vi "Autonomous.vi"   [LabVIEW 2018]
doc: "This VI starts when autonomous period begins, and will automatically be terminated when it ends. You can carry out timed or sensor driven operations directly to I/O or to subsystems without needing to return to the caller."
uses:
  <vilib>/Rock Robotics/WPI/Solenoid/WPI_SolenoidValue.ctl
  <vilib>/Rock Robotics/WPI/Utilities/WPI_GetSetVariantRefNum.vi
  <vilib>/Rock Robotics/Network Tables/NT Read String.vi
  Framework/Robot Global Data.vi
types:
  T1 = typedef "WPI_JoystickDevRef.ctl" = cluster{"Device":T2}
  T2 = typedef "WPI_JoystickDeviceEnum.ctl" = enum16{"USB 0", "USB 1", "USB 2", "USB 3", "USB 4", "USB 5"}
  T3 = typedef "WPI_SolenoidValue.ctl" = enum16{"Off", "On", "Forward", "Reverse"}
  T4 = typedef "Command Status Info.ctl" = cluster{"Name":string, "Status":T5, "notifier out":T6}
  T5 = typedef "Completion Status.ctl" = enum16{"Successful", "Aborted", "Incomplete"}
  T6 = typedef "Completion Notifier.ctl" = refnum<notifier>
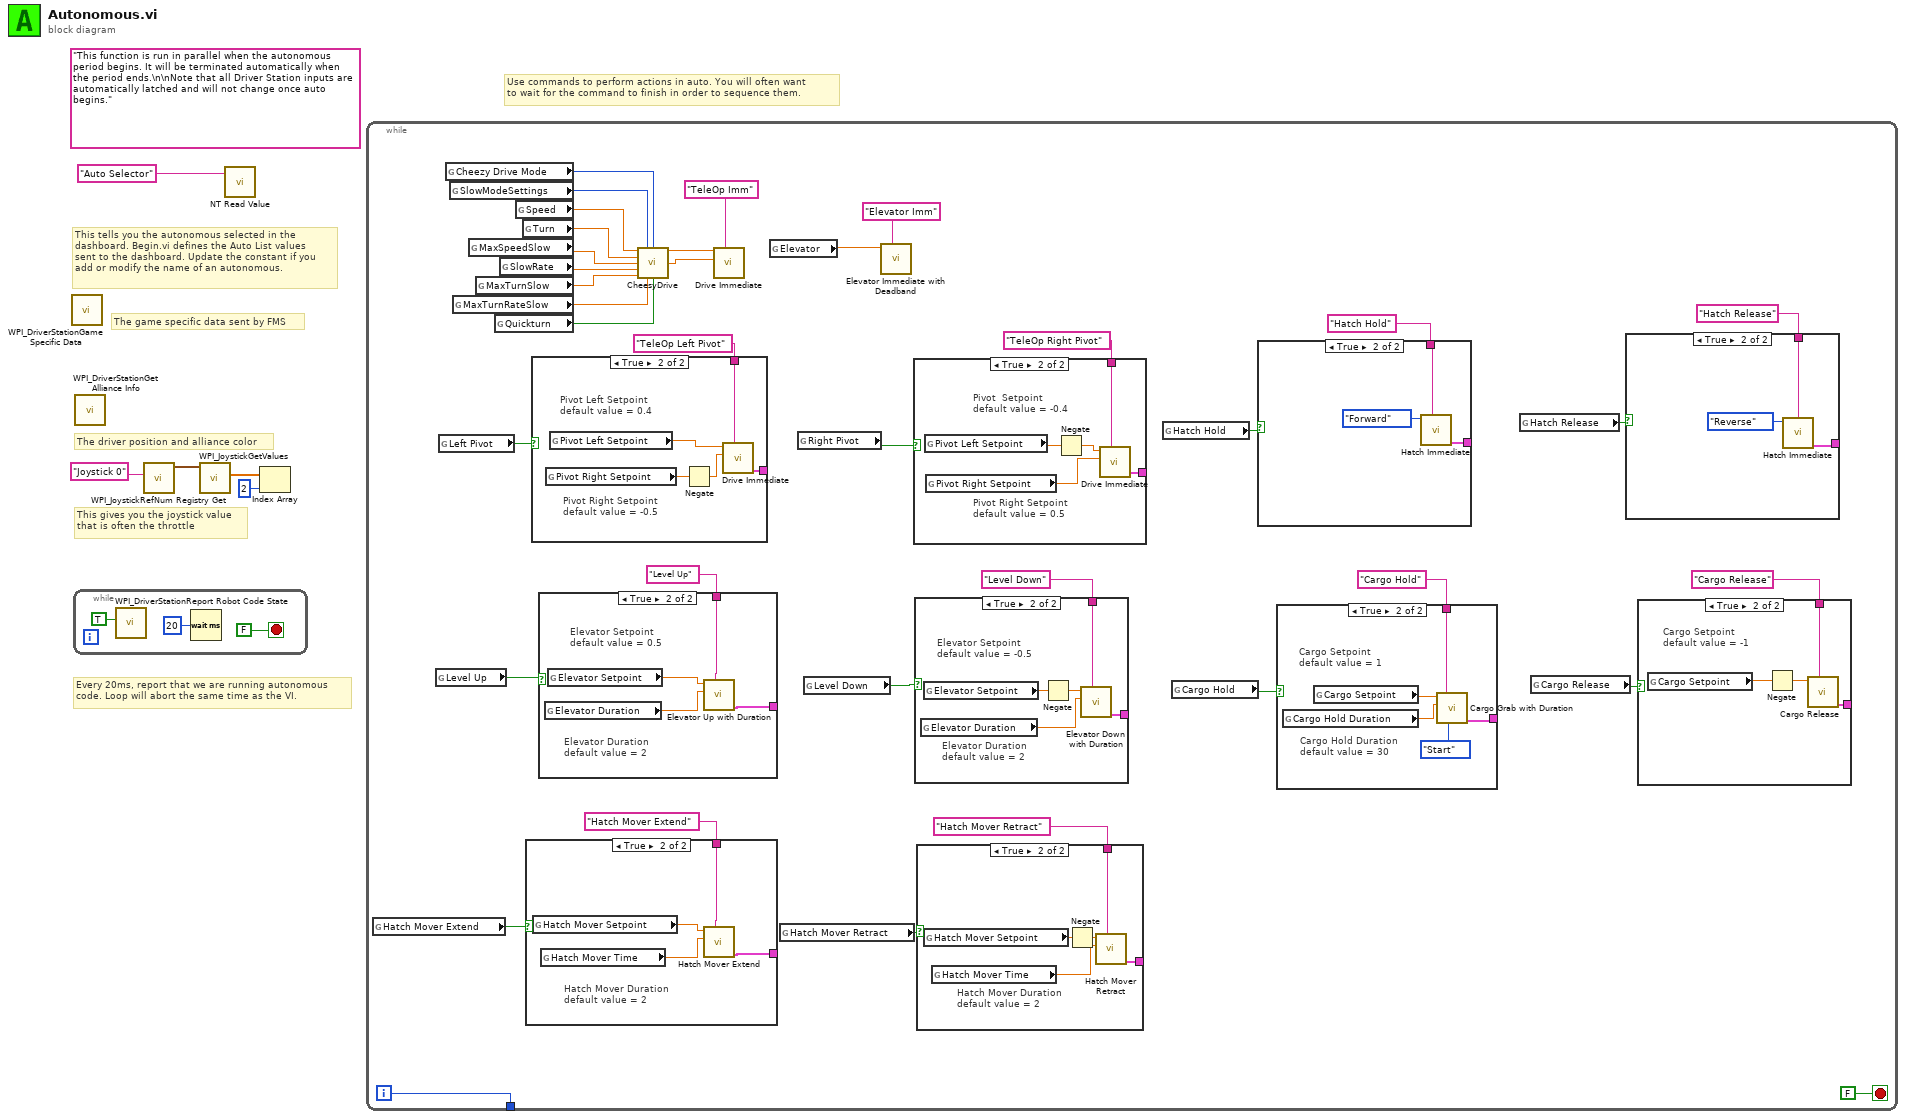
[diagram p0: block diagram]
diagram:
  (unwired) "This function is run in parallel when the autonomous period begins. It will be terminated automatically when the period ends.\n\nNote that all Driver Station inputs are automatically latched and will not change once auto begins."
  # "The game specific data sent by FMS"
  # "This tells you the autonomous selected in the \ndashboard. Begin.vi defines the Auto List values\nsent to the dashboard. Update the constant if you\nadd or modify the name of an autonomous."
  # "Every 20ms, report that we are running autonomous\ncode. Loop will abort the same time as the VI."
  # "This gives you the joystick value\nthat is often the throttle"
  # "Use commands to perform actions in auto. You will often want\nto wait for the command to finish in order to sequence them."
  # "The driver position and alliance color"
  n1 = call <vilib>:"WPI_DriverStationGame Specific Data.vi"() -> ()  [unwired: 11 in, 1 out]
  n2 = while {
    stop <- FALSE stop-if-true
    n3 = call <vilib>:"WPI_DriverStationReport Robot Code State.vi"("Autonomous"=TRUE) -> ()  [unwired: 10 in, 1 out]
    n4 = Wait (ms)(milliseconds to wait=u32 20) -> ()  [unwired: 1 out]
  }
  n5 = call <vilib>:"WPI_DriverStationGet Alliance Info.vi"() -> ()  [unwired: 12 out]
  n6 = call <vilib>:"WPI_JoystickRefNum Registry Get.vi"("refnum name"="Joystick 0") -> ("JoystickDevRef"=w4:T1)  [unwired: 1 in, 9 out]
  n7 = call <vilib>:"WPI_JoystickGetValues.vi"("JoystickDevRef"=w4) -> ("Axes"=w3:dbl[])  [unwired: 6 in, 4 out]
  n8 = call-poly <vilib>:"NT Read Value.vi"("Name"="Auto Selector") -> ()  [unwired: 9 in, 2 out]
  n9 = Index Array(array=w3, index=2) -> ()  [unwired: 1 out]
  n10 = while {
    tunnel: [w9] -> _
    i -> [w9]
    stop <- FALSE stop-if-true
    n11 = global read "Robot Global Data.vi" "Hatch Mover Extend"() -> (w16:bool)
    n12 = global read "Robot Global Data.vi" "Level Up"() -> (w21:bool)
    n13 = global read "Robot Global Data.vi" "Left Pivot"() -> (w27:bool)
    n14 = global read "Robot Global Data.vi" "Cheezy Drive Mode"() -> (w41:u32)
    n15 = global read "Robot Global Data.vi" "SlowModeSettings"() -> (w31:i32)
    n16 = global read "Robot Global Data.vi" "MaxTurnRateSlow"() -> (w33:dbl)
    n17 = global read "Robot Global Data.vi" "MaxSpeedSlow"() -> (w36:dbl)
    n18 = global read "Robot Global Data.vi" "MaxTurnSlow"() -> (w34:dbl)
    n19 = global read "Robot Global Data.vi" "Quickturn"() -> (w32:bool)
    n20 = global read "Robot Global Data.vi" "SlowRate"() -> (w35:dbl)
    n21 = global read "Robot Global Data.vi" "Speed"() -> (w38:dbl)
    n22 = global read "Robot Global Data.vi" "Turn"() -> (w37:dbl)
    n23 = case shown="True" w16 {
      tunnel: [_ w62] -> _
      tunnel: "Hatch Mover Extend" ("Description") -> [_ w61]
      frame False {
      }
      frame True {
        # "Hatch Mover Duration\ndefault value = 2"
        n24 = global read "Robot Global Data.vi" "Hatch Mover Setpoint"() -> (w60:dbl)
        n25 = global read "Robot Global Data.vi" "Hatch Mover Time"() -> (w59:dbl)
        n26 = call "Hatch Mover Extend.vi"("Description"=w61, "Duration (s)"=w59, "Setpoint"=w60) -> ("Command Info Out"=w62:T4)  [unwired: 8 in]
      }
    }
    n27 = case shown="True" w27 {
      tunnel: [_ w87] -> _
      tunnel: "TeleOp Left Pivot" ("Description") -> [_ w86]
      frame False {
      }
      frame True {
        # "Pivot Right Setpoint\ndefault value = -0.5"
        # "Pivot Left Setpoint\ndefault value = 0.4"
        n28 = global read "Robot Global Data.vi" "Pivot Right Setpoint"() -> (w84:dbl)
        n29 = global read "Robot Global Data.vi" "Pivot Left Setpoint"() -> (w85:dbl)
        n30 = Negate(x=w84) -> (-x=w83:dbl)
        n31 = call "Drive Immediate.vi"("Description"=w86, "Right Setpoint"=w83, "Left Setpoint"=w85) -> ("Command Info Out"=w87:T4)  [unwired: 8 in]
      }
    }
    n32 = case shown="True" w21 {
      tunnel: [_ w71] -> _
      tunnel: "Level Up" ("Description") -> [_ w70]
      frame False {
      }
      frame True {
        # "Elevator Setpoint\ndefault value = 0.5"
        # "Elevator Duration\ndefault value = 2"
        n33 = global read "Robot Global Data.vi" "Elevator Duration"() -> (w68:dbl)
        n34 = global read "Robot Global Data.vi" "Elevator Setpoint"() -> (w69:dbl)
        n35 = call "Elevator Up with Duration.vi"("Description"=w70, "Duration (s)"=w68, "Setpoint"=w69) -> ("Command Info Out"=w71:T4)  [unwired: 8 in]
      }
    }
    n36 = call "CheesyDrive.vi"("Throttle"=w38, "SlowModeSettings"=w31, "SlowMode"=w41, "Wheel"=w37, "MaxSpeedSlow"=w36, "SlowRate"=w35, "MaxTurnSlow"=w34, "MaxTurnRateSlow"=w33, "Quickturn"=w32) -> ("Left PWM"=w40:dbl, "Right PWM"=w39:dbl)  [unwired: 5 in]
    n37 = call "Drive Immediate.vi"("Description"="TeleOp Imm", "Right Setpoint"=w39, "Left Setpoint"=w40) -> ()  [unwired: 8 in, 1 out]
    n38 = global read "Robot Global Data.vi" "Elevator"() -> (w43:dbl)
    n39 = global read "Robot Global Data.vi" "Hatch Mover Retract"() -> (w17:bool)
    n40 = global read "Robot Global Data.vi" "Right Pivot"() -> (w28:bool)
    n41 = global read "Robot Global Data.vi" "Level Down"() -> (w20:bool)
    n42 = call "Elevator Immediate with Deadband.vi"("Description"="Elevator Imm", "Setpoint"=w43) -> ()  [unwired: 9 in, 1 out]
    n43 = case shown="True" w28 {
      tunnel: [_ w82] -> _
      tunnel: "TeleOp Right Pivot" ("Description") -> [_ w81]
      frame False {
      }
      frame True {
        # "Pivot Right Setpoint\ndefault value = 0.5"
        # "Pivot  Setpoint\ndefault value = -0.4"
        n44 = global read "Robot Global Data.vi" "Pivot Left Setpoint"() -> (w79:dbl)
        n45 = global read "Robot Global Data.vi" "Pivot Right Setpoint"() -> (w80:dbl)
        n46 = Negate(x=w79) -> (-x=w78:dbl)
        n47 = call "Drive Immediate.vi"("Description"=w81, "Right Setpoint"=w80, "Left Setpoint"=w78) -> ("Command Info Out"=w82:T4)  [unwired: 8 in]
      }
    }
    n48 = case shown="True" w20 {
      tunnel: "Level Down" ("Description") -> [_ w67]
      tunnel: [_ w66] -> _
      frame False {
      }
      frame True {
        # "Elevator Duration\ndefault value = 2"
        # "Elevator Setpoint\ndefault value = -0.5"
        n49 = global read "Robot Global Data.vi" "Elevator Duration"() -> (w64:dbl)
        n50 = global read "Robot Global Data.vi" "Elevator Setpoint"() -> (w65:dbl)
        n51 = Negate(x=w65) -> (-x=w63:dbl)
        n52 = call "Elevator Down with Duration.vi"("Description"=w67, "Duration (s)"=w64, "Setpoint"=w63) -> ("Command Info Out"=w66:T4)  [unwired: 8 in]
      }
    }
    n53 = case shown="True" w17 {
      tunnel: "Hatch Mover Retract" ("Description") -> [_ w58]
      tunnel: [_ w57] -> _
      frame False {
      }
      frame True {
        # "Hatch Mover Duration\ndefault value = 2"
        n54 = global read "Robot Global Data.vi" "Hatch Mover Setpoint"() -> (w56:dbl)
        n55 = global read "Robot Global Data.vi" "Hatch Mover Time"() -> (w55:dbl)
        n56 = Negate(x=w56) -> (-x=w54:dbl)
        n57 = call "Hatch Mover Retract.vi"("Description"=w58, "Duration (s)"=w55, "Setpoint"=w54) -> ("Command Info Out"=w57:T4)  [unwired: 8 in]
      }
    }
    n58 = global read "Robot Global Data.vi" "Hatch Hold"() -> (w23:bool)
    n59 = global read "Robot Global Data.vi" "Cargo Hold"() -> (w12:bool)
    n60 = case shown="True" w23 {
      tunnel: "Hatch Hold" ("Description") -> [_ w77]
      tunnel: [_ w76] -> _
      frame False {
      }
      frame True {
        n61 = call "Hatch Immediate.vi"("Description"=w77, "Hatch Action"=WPI_SolenoidValue."Forward") -> ("Command Info Out"=w76:T4)  [unwired: 9 in]
      }
    }
    n62 = case shown="True" w12 {
      tunnel: [_ w53] -> _
      tunnel: "Cargo Hold" ("Description") -> [_ w52]
      frame False {
      }
      frame True {
        # "Cargo Hold Duration\ndefault value = 30"
        # "Cargo Setpoint\ndefault value = 1"
        n63 = global read "Robot Global Data.vi" "Cargo Hold Duration"() -> (w49:dbl)
        n64 = global read "Robot Global Data.vi" "Cargo Setpoint"() -> (w51:dbl)
        n65 = call "Cargo Grab with Duration.vi"("Synchronization"=enum16{"Start", "Wait"}."Start", "Description"=w52, "Duration (s)"=w49, "Setpoint"=w51) -> ("Command Info Out"=w53:T4)  [unwired: 7 in]
      }
    }
    n66 = global read "Robot Global Data.vi" "Hatch Release"() -> (w24:bool)
    n67 = global read "Robot Global Data.vi" "Cargo Release"() -> (w11:bool)
    n68 = case shown="True" w24 {
      tunnel: "Hatch Release" ("Description") -> [_ w74]
      tunnel: [_ w73] -> _
      frame False {
      }
      frame True {
        n69 = call "Hatch Immediate.vi"("Description"=w74, "Hatch Action"=WPI_SolenoidValue."Reverse") -> ("Command Info Out"=w73:T4)  [unwired: 9 in]
      }
    }
    n70 = case shown="True" w11 {
      tunnel: [_ w48] -> _
      tunnel: "Cargo Release" ("Description") -> [_ w47]
      frame False {
      }
      frame True {
        # "Cargo Setpoint\ndefault value = -1"
        n71 = global read "Robot Global Data.vi" "Cargo Setpoint"() -> (w46:dbl)
        n72 = Negate(x=w46) -> (-x=w45:dbl)
        n73 = call "Cargo Release.vi"("Description"=w47, "Setpoint"=w45) -> ("Command Info Out"=w48:T4)  [unwired: 9 in]
      }
    }
  }
